vi "optionsAcq_PDTemperatureMode.vi"(0 "reference":refnum<class "OSA300.lvclass">, 2 "PD sensitivity mode":T1, 5 "error in (no error)":errorcluster, 9 "read/write":enum16{"read", "write"}(ring)) -> (14 "duplicate reference":refnum<class "OSA300.lvclass">, 16 "PD sensitivity mode out":T1, 18 "PD senseMode implemented":bool, 19 "error out":errorcluster)   [LabVIEW 2010, in "OSA300.lvclass"]
doc: "The OSA optical detectors in some models are cooled to improve the noise floor, (typically cooled at -30 degrees C for a reduction of thermal noise). However the cooling also restricts the upper wavelength range which is why a warm detector temperature mode can be selected to extend the range.\n[OSA200]"
uses:
  OSA300.lvclass
  _misc/Thorlabs_FTS_misc.llb/PDTemperatureMode.ctl
  OSA300.lvclass/OSA300.ctl
  OSA.lvclass
  _OSAchannel_class/OSAchannel.lvclass
  OSA20X_misc.lvlib
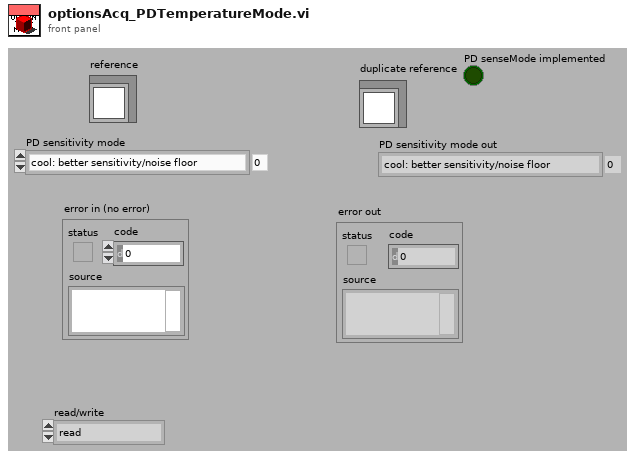
[diagram p1: front panel]
types:
  T1 = typedef "OSA20X_misc.lvlib/PDTemperatureMode.ctl" = enum16{"cool: better sensitivity/noise floor", "warm: extended wl range"}
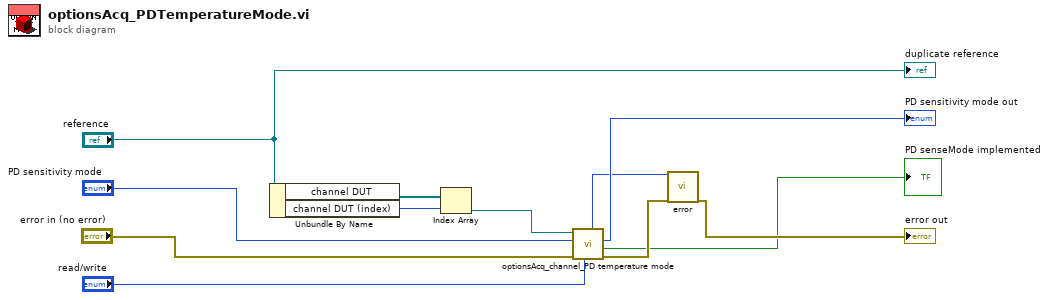
[diagram p0: block diagram]
diagram:
  n1 = Unbundle By Name("reference") -> ("channel DUT"=w12:refnum<class "OSAchannel.lvclass">[], "channel DUT (index)"=w11:i32)
  n2 = Index Array(array=w12, index=w11) -> (element=w10:refnum<class "OSAchannel.lvclass">)
  n3 = call "optionsAcq_channel_PD temperature mode.vi"("read/write"="read/write", "error in (no error)"="error in (no error)", "PD sensitivity mode write"="PD sensitivity mode", "OSAchannel in"=w10) -> ("error out"=w6:errorcluster, "channel.temp Variable"=→"PD senseMode implemented":bool, "PD sensitivity mode out"=→"PD sensitivity mode out":T1, "status FTSLib"=w2:i32)  [unwired: 3 in, 1 out]
  n4 = call "error.vi"("result code"=w2, "error in (no error)"=w6) -> ("error out"=→"error out":errorcluster)  [unwired: 15 in, 2 out]
  "duplicate reference" <- "reference"
